vi "Generic command handler.vi"(8 "error in (no error)":errorcluster, 10 "Message in":refnum<class "GenericMessage.lvclass">, 11 "Piezo in":refnum<class "Piezo.lvclass">) -> (0 "error out":errorcluster, 2 "value":string, 3 "Piezo out":refnum<class "Piezo.lvclass">)   [LabVIEW 2012, in "Piezo.lvclass"]
doc: "The generic_command_handler processes the command 'generic'. Commands which are not part of the predefined list of commands fall under the 'generic' command for special activity."
uses:
  Piezo.lvclass
  <vilib>/Distrio/Murmex/GenericMessage/GenericMessage.lvclass
  <vilib>/Distrio/Murmex/Murmex/Murmex.lvclass
  Piezo.lvclass/Piezo.ctl
  <vilib>/Distrio/Murmex/ProceedMessage/ProceedMessage.lvclass
  <vilib>/DAQmx/write.llb/DAQmx Write (Analog DBL 1Chan 1Samp).vi
  <vilib>/Distrio/Murmex/Message/Message.lvclass
panel:
  # "This method is called when the GENERIC\ntrigger is sent. \n\nOverride this method when your component needs to\nrespond to this trigger. \n\nCall parent for proper implementation"
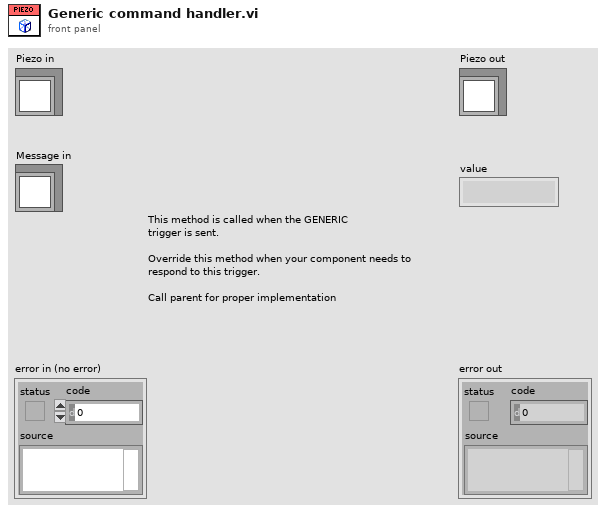
[diagram p1: front panel]
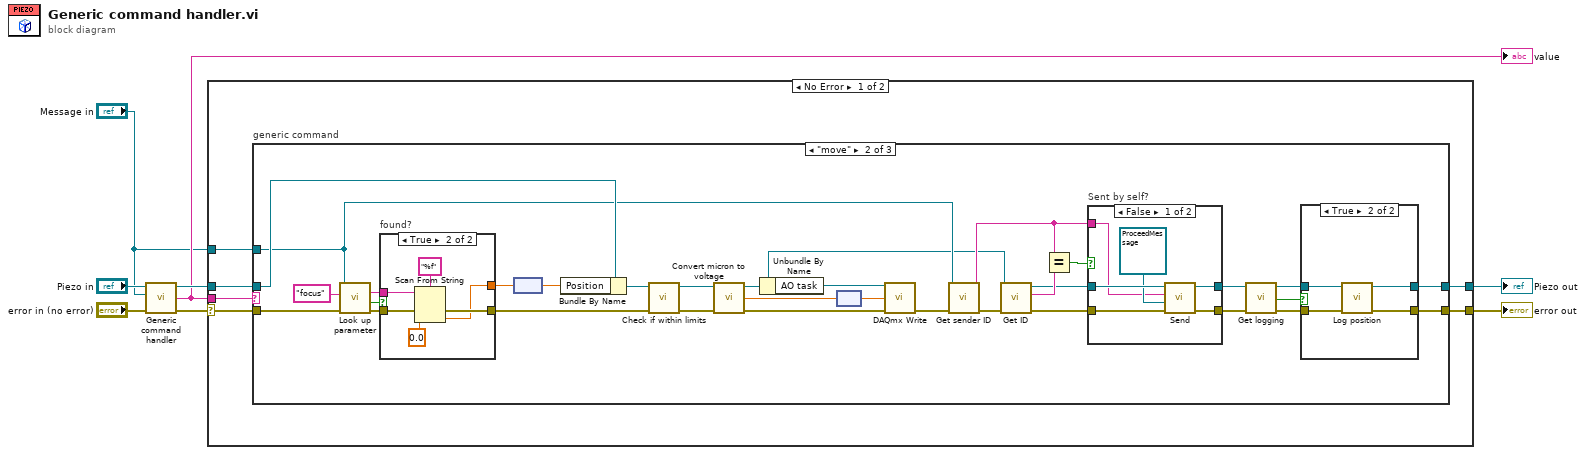
[diagram p0: block diagram]
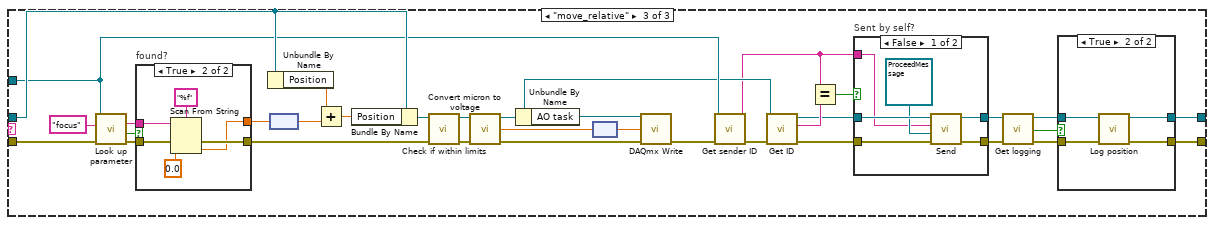
[diagram p6: hidden frame]
diagram:
  n1 = call-parent "Generic command handler.vi"("error in (no error)"="error in (no error)", "Message in"="Message in", "Murmex in"="Piezo in") -> ("error out"=w6:errorcluster, "value"=w2:string, "Murmex out"=w3:refnum<class "Piezo.lvclass">)  [unwired: 6 in]
  "value" <- w2
  n2 = case shown="No Error" w6 {
    selector: w6 -> [w12 w125]
    tunnel: w2 -> [w14 _]
    tunnel: [w13 w125] -> w5
    tunnel: [w11 w126] -> w4
    tunnel: w3 -> [w10 w126]
    tunnel: "Message in" -> [w9 _]
    frame No Error {
      n3 = case "generic command" shown="\"move\"" w14 {
        tunnel: [w16 w21 w74] -> w13
        tunnel: w12 -> [w16 w48 w103]
        tunnel: [w15 w22 w75] -> w11
        tunnel: w10 -> [w15 w42 w93]
        tunnel: w9 -> [_ w29 w89]
        frame Default {
        }
        frame "move" {
          n4 = call <vilib>:"Look up parameter.vi"("error in (no error)"=w48, "name"="focus", "Message in"=w29) -> ("error out"=w45:errorcluster, "found?"=w46:bool, "key"=w44:string)  [unwired: 5 in, 1 out]
          n5 = case "found?" shown="True" w46 {
            tunnel: w45 -> [w63 w68]
            tunnel: w44 -> [_ w67]
            tunnel: [w63 w65] -> w17
            tunnel: [_ w64] -> w43
            frame False {
            }
            frame True {
              n6 = Scan From String(format string="%f", input string=w67, error in=w68, default 1=0.0 ("default value 1")) -> (error out=w65:errorcluster, output 1=w64:dbl)  [unwired: 1 in, 2 out]
            }
          }
          n7 = node(w43) -> (w41:dbl[unit])
          n8 = Bundle By Name(cluster=w42, "Position"=w41) -> (w20:refnum<class "Piezo.lvclass">)
          n9 = call-dynamic "Check if within limits.vi"("error in (no error)"=w17, "Piezo in"=w20) -> ("error out"=w18:errorcluster, "Piezo out"=w19:refnum<class "Piezo.lvclass">)  [unwired: 7 in, 1 out]
          n10 = call-dynamic "Convert micron to voltage.vi"("error in (no error)"=w18, "Piezo in"=w19) -> ("error out"=w40:errorcluster, "Output voltage"=w38:dbl[unit], "Piezo out"=w28:refnum<class "Piezo.lvclass">)  [unwired: 7 in]
          n11 = Unbundle By Name(w28) -> ("AO task"=w39:refnum<k21>)
          n12 = node(w38) -> (w37:dbl)
          n13 = call-poly <vilib>:"DAQmx Write.vi"("task/channels in"=w39, "data"=w37, "error in"=w40) -> ("error out"=w30:errorcluster)  [unwired: 10 in, 2 out]
          n14 = call <vilib>:"Get sender ID.vi"("error in (no error)"=w30, "Message in"=w29) -> ("error out"=w36:errorcluster, "sender"=w31:string)  [unwired: 7 in, 1 out]
          n15 = call <vilib>:"Get ID.vi"("error in (no error)"=w36, "Murmex in"=w28) -> ("error out"=w33:errorcluster, "component id"=w35:string, "Murmex out"=w32:refnum<class "Piezo.lvclass">)  [unwired: 7 in]
          n16 = Equal?(x=w31, y=w35) -> (x = y?=w34:bool)
          n17 = case "Sent by self?" shown="False" w34 {
            tunnel: [w57 w62] -> w26
            tunnel: w33 -> [w60 w62]
            tunnel: [w58 w61] -> w27
            tunnel: w32 -> [w59 w61]
            tunnel: w31 -> [w55 _]
            frame False {
              n18 = call <vilib>:"Send.vi"("error in (no error)"=w60, "Message"=refnum<class "ProceedMessage.lvclass"> refnum ("ProceedMessage"), "recipient"=w55, "Murmex in"=w59) -> ("error out"=w57:errorcluster, "Murmex out"=w58:refnum<class "Piezo.lvclass">)  [unwired: 6 in]
            }
            frame True {
            }
          }
          n19 = call-dynamic "Get logging.vi"("error in (no error)"=w26, "Piezo in"=w27) -> ("error out"=w24:errorcluster, "logging?"=w25:bool, "Piezo out"=w23:refnum<class "Piezo.lvclass">)  [unwired: 7 in]
          n20 = case shown="True" w25 {
            tunnel: w24 -> [w49 w54]
            tunnel: w23 -> [w50 w53]
            tunnel: [w50 w52] -> w22
            tunnel: [w49 w51] -> w21
            frame False {
            }
            frame True {
              n21 = call-dynamic "Log position.vi"("error in (no error)"=w54, "Piezo in"=w53) -> ("error out"=w51:errorcluster, "Piezo out"=w52:refnum<class "Piezo.lvclass">)  [unwired: 8 in]
            }
          }
        }
        frame "move_relative" {
          n22 = call <vilib>:"Look up parameter.vi"("error in (no error)"=w103, "name"="focus", "Message in"=w89) -> ("error out"=w100:errorcluster, "found?"=w101:bool, "key"=w99:string)  [unwired: 5 in, 1 out]
          n23 = case "found?" shown="True" w101 {
            tunnel: w100 -> [w118 w123]
            tunnel: w99 -> [_ w122]
            tunnel: [w118 w120] -> w71
            tunnel: [_ w119] -> w98
            frame False {
            }
            frame True {
              n24 = Scan From String(format string="%f", input string=w122, error in=w123, default 1=0.0 ("default value 1")) -> (error out=w120:errorcluster, output 1=w119:dbl)  [unwired: 1 in, 2 out]
            }
          }
          n25 = Unbundle By Name(w93) -> ("Position"=w92:dbl[unit])
          n26 = node(w98) -> (w91:dbl[unit])
          n27 = Add(x=w92, y=w91) -> (x+y=w90:dbl[unit])
          n28 = Bundle By Name(cluster=w93, "Position"=w90) -> (w73:refnum<class "Piezo.lvclass">)
          n29 = call-dynamic "Check if within limits.vi"("error in (no error)"=w71, "Piezo in"=w73) -> ("error out"=w70:errorcluster, "Piezo out"=w72:refnum<class "Piezo.lvclass">)  [unwired: 7 in, 1 out]
          n30 = call-dynamic "Convert micron to voltage.vi"("error in (no error)"=w70, "Piezo in"=w72) -> ("error out"=w97:errorcluster, "Output voltage"=w95:dbl[unit], "Piezo out"=w86:refnum<class "Piezo.lvclass">)  [unwired: 7 in]
          n31 = Unbundle By Name(w86) -> ("AO task"=w96:refnum<k21>)
          n32 = node(w95) -> (w94:dbl)
          n33 = call-poly <vilib>:"DAQmx Write.vi"("task/channels in"=w96, "data"=w94, "error in"=w97) -> ("error out"=w87:errorcluster)  [unwired: 10 in, 2 out]
          n34 = call <vilib>:"Get sender ID.vi"("error in (no error)"=w87, "Message in"=w89) -> ("error out"=w88:errorcluster, "sender"=w81:string)  [unwired: 7 in, 1 out]
          n35 = call <vilib>:"Get ID.vi"("error in (no error)"=w88, "Murmex in"=w86) -> ("error out"=w83:errorcluster, "component id"=w85:string, "Murmex out"=w82:refnum<class "Piezo.lvclass">)  [unwired: 7 in]
          n36 = Equal?(x=w81, y=w85) -> (x = y?=w84:bool)
          n37 = case "Sent by self?" shown="False" w84 {
            tunnel: [w112 w117] -> w76
            tunnel: w83 -> [w115 w117]
            tunnel: [w113 w116] -> w77
            tunnel: w82 -> [w114 w116]
            tunnel: w81 -> [w110 _]
            frame False {
              n38 = call <vilib>:"Send.vi"("error in (no error)"=w115, "Message"=refnum<class "ProceedMessage.lvclass"> refnum ("ProceedMessage"), "recipient"=w110, "Murmex in"=w114) -> ("error out"=w112:errorcluster, "Murmex out"=w113:refnum<class "Piezo.lvclass">)  [unwired: 6 in]
            }
            frame True {
            }
          }
          n39 = call-dynamic "Get logging.vi"("error in (no error)"=w76, "Piezo in"=w77) -> ("error out"=w79:errorcluster, "logging?"=w80:bool, "Piezo out"=w78:refnum<class "Piezo.lvclass">)  [unwired: 7 in]
          n40 = case shown="True" w80 {
            tunnel: w79 -> [w104 w109]
            tunnel: w78 -> [w105 w108]
            tunnel: [w105 w107] -> w75
            tunnel: [w104 w106] -> w74
            frame False {
            }
            frame True {
              n41 = call-dynamic "Log position.vi"("error in (no error)"=w109, "Piezo in"=w108) -> ("error out"=w106:errorcluster, "Piezo out"=w107:refnum<class "Piezo.lvclass">)  [unwired: 8 in]
            }
          }
        }
      }
    }
    frame Error {
    }
  }
  "error out" <- w5
  "Piezo out" <- w4
